vi "_Update Shutting Down.vi"(4 "error in (no error)":errorcluster, 7 "Fault":bool) -> (0 "error Out":errorcluster, 1 "Cancelled":bool, 2 "Error":bool, 3 "InstrState":T1=enum."Fault")   [LabVIEW 2012]
uses:
  Type/_RT Instrument State.ctl
  Type/_LCD Line1 Msg.ctl
  Type/_LCD Line2 Msg.ctl
  Type/_RT LED Num.ctl
  Type/_LED States.ctl
  Type/_Pump Parameter.ctl
  Type/_RW Status.ctl
  _RT Global.vi
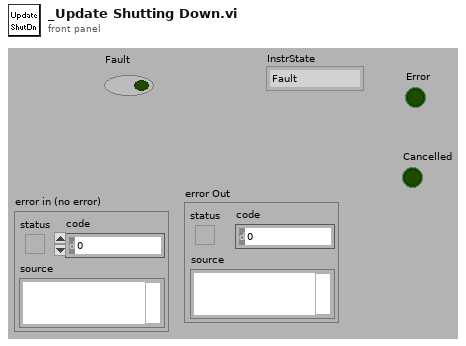
[diagram p1: front panel]
types:
  T1 = typedef "_RT Instrument State.ctl" = enum16{"Initializing", "Mass Spectrometer is Off", "Starting Up", "Turning Power Off", "Going to Standby", "Roughing Pump Ready", "Turning Turbo Off", "Turbo Startup", "Turbopump Ready", "Checking Vacuum", "Going to Ready", "Ready", "Running", "Source Standby", "Lost Communication", "Shutting Down", "Fault", "24V Standby", "Go to 24V Standby", "Turbopump Ready-Waiting"}
  T2 = typedef "_RT LED Num.ctl" = enum8{"ReadKey", "ClearKeyBuffer", "ClearLCD", "BacklightOn"}
  T3 = typedef "_Pump Parameter.ctl" = enum16{"Turn Pump Motor On", "Turn Pump Motor Off", "Read Pump Oil Deficiency", "Read Rotation Switch Point Attained", "Read Ele. Drive Over Temperature", "Read Pump Over Temperature", "Read Set Rotation Speed Attained", "Read Turbopump Accelerates", "Read Actual Rotation Speed in Hz", "Read Motor Current in A", "Read Operating Hours in h", "Read Motor Voltage in V", "Read Motor Power in W", "Set Rotation Speed Switchpoint in %", "Clear Error", "Read Error Code", "Read Bearing Temperature", "Read Hardware Version", "Read Firmware Version", "Read Operating Hours (Drive)", "Read Rotational Speed (rpm)", "Read Power Stage Temperature", "Read Electronics Temperature", "Read Upper Pump Temperature", "Read Motor Temperature", "Read Error Code History, 1", "Read Error Code History, 2", "Read Error Code History, 3", "Read Error Code History, 4", "Read Error Code History, 5", "Read Error Code History, 6", "Read Error Code History, 7", "Read Error Code History, 8", "Read Error Code History, 9", "Read Error Code History, 10"}
  T4 = typedef "_LED States.ctl" = enum8{"Idle", "Solid B", "Solid R", "Solid P", "Off B", "Off R", "Off P", "Off BRP", "Off RP", "Flash R&P", "Flash P"}
  T5 = typedef "_RW Status.ctl" = enum8{"Done", "Do Read", "Do Write", "Set Latch1", "Set Latch2", "Set Latch3", "Set Latch4", "RP ON", "EL ON", "Serial Send", "Set LC Out", "Get LC In", "Read VAC", "Table Test", "Get Interlock", "Do Read2", "Do Write2"}
  T6 = typedef "_LCD Line2 Msg.ctl" = u16
  T7 = typedef "_LCD Line1 Msg.ctl" = u16
  T8 = typedef "_RT Startup Options.ctl" = cluster{"Door":bool, "Curtain":bool, "Pressure":bool, "Turbo":bool, "SysPoll":bool, "GasFlag":bool}
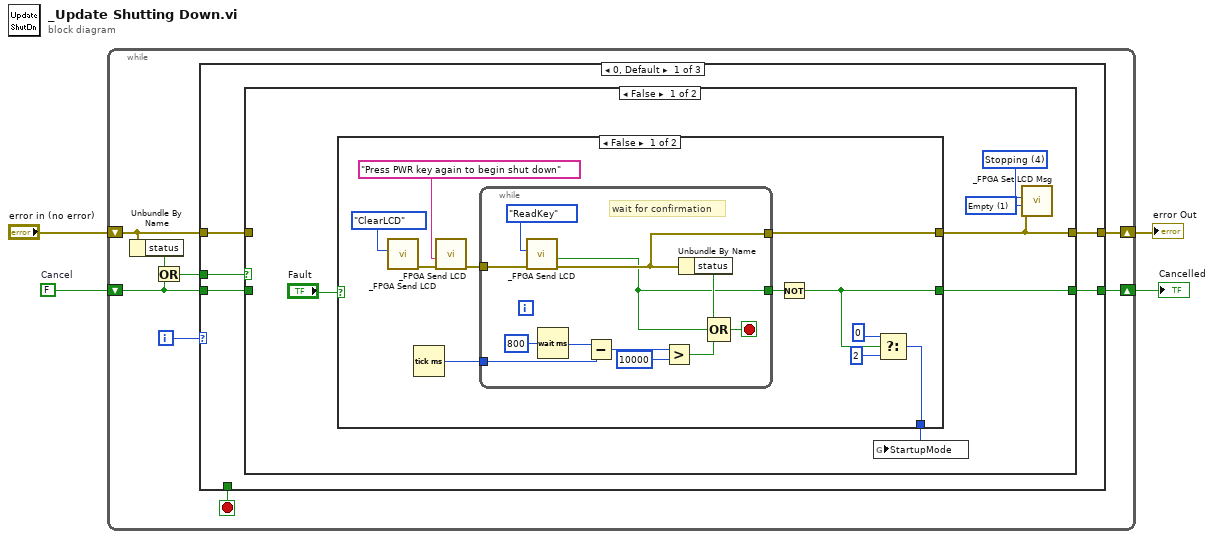
[diagram p0: block diagram]
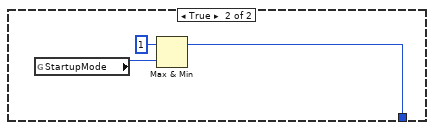
[diagram p2: hidden frame]
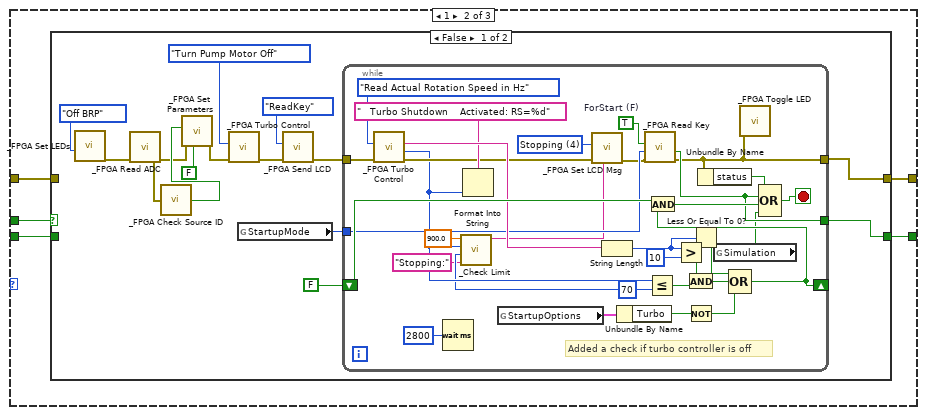
[diagram p4: hidden frame]
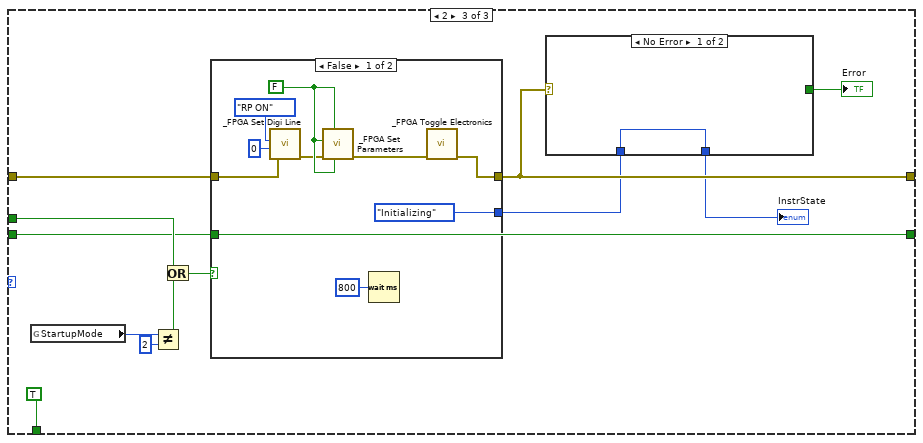
[diagram p6: hidden frame]
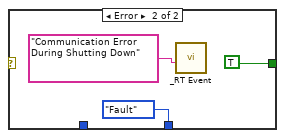
[diagram p7: hidden frame]
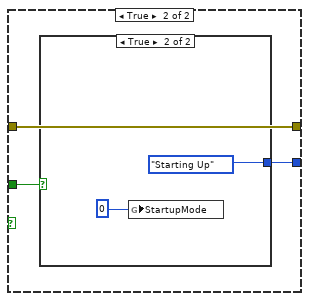
[diagram p8: hidden frame]
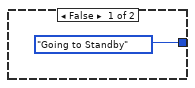
[diagram p9: hidden frame]
diagram:
  w3 = FALSE  # Cancel
  n1 = while {
    shift-right: [w6] -> w2
    shift-left: "error in (no error)" -> [w11]
    shift-right: [w5] -> w1
    shift-left: w3 -> [w10]
    i -> [w8]
    stop <- w7 stop-if-true
    n2 = Unbundle By Name(w11) -> ("status"=w12:bool)
    n3 = Or(x=w12, y=w10) -> (x .or. y?=w9:bool)
    n4 = case shown="0, Default" w8 {
      tunnel: w11 -> [w16 w56 w116]
      tunnel: w10 -> [w14 w54 w105]
      tunnel: w9 -> [w17 w52 w111]
      tunnel: [_ _ TRUE] -> w7
      tunnel: [w15 w55 w114] -> w6
      tunnel: [w13 w53 w105] -> w5
      frame 0, Default {
        n5 = case shown="False" w17 {
          tunnel: w16 -> [_ w51]
          tunnel: [w18 w51] -> w15
          tunnel: w14 -> [_ w50]
          tunnel: [w22 w50] -> w13
          frame False {
            w19 = T6 1 items=["Same", "Empty", "VacFail", "Cancel", "CheckGas", "EleFail", "Probe1Fail", "Probe2Fail", "HeaterFail", "DoorOpen", "CheckComm", "PressStart"] ("Line2Msg (same)")
            w20 = T7 4 items=["Same", "Empty", "Connected", "Starting", "Stopping", "Action", "On", "Service", "Call", "Acquiring", "Source"] ("Line1Msg (same)")
            n6 = case shown="False" "Fault" {
              tunnel: [w33 _] -> w18
              tunnel: [w30 _] -> w22
              tunnel: [w28 w47] -> w21
              frame False {
                n7 = call "_FPGA Send LCD.vi"("Command"=_RT_LED_Num."ClearLCD" ("LED#")) -> ("error out"=w27:errorcluster)  [unwired: 4 in, 3 out]
                n8 = Tick Count (ms)() -> (millisecond timer value=w34:u32)
                n9 = call "_FPGA Send LCD.vi"("error in (no error)"=w27, "Message"="Press PWR key again to begin shut down" ("Command")) -> ("error out"=w25:errorcluster)  [unwired: 3 in, 3 out]
                n10 = while {
                  tunnel: w25 -> [w38]
                  tunnel: [w37] -> w33
                  tunnel: w34 -> [w42]
                  tunnel: [w35] -> w32
                  stop <- w45 stop-if-true
                  # "wait for confirmation"
                  n11 = call "_FPGA Send LCD.vi"("error in (no error)"=w38, "Command"=_RT_LED_Num."ReadKey" ("LED#")) -> ("error out"=w37:errorcluster, "Key Pressed"=w35:bool)  [unwired: 3 in, 2 out]
                  n12 = Wait (ms)(milliseconds to wait=u32 800) -> (millisecond timer value=w43:u32)
                  n13 = Subtract(x=w43, y=w42) -> (x-y=w41:u32)
                  n14 = Greater?(x=w41, y=u32 10000) -> (0:w36:bool)
                  n15 = Unbundle By Name(w37) -> ("status"=w44:bool)
                  n16 = Compound Arithmetic op=OR(w44, w35, w36) -> (w45:bool)
                }
                n17 = Not(x=w32) -> (.not. x?=w30:bool)
                n18 = Select(t=u8 0 ("f"), s=w30, f=u8 2) -> (s? t:f=w28:u8)
              }
              frame True {
                n19 = global read "_RT Global.vi" "StartupMode"() -> (w49:u8)
                n20 = Max & Min(x=u8 1, y=w49) -> (max(x,y)=w47:u8)  [unwired: 1 out]
              }
            }
            n21 = global write "_RT Global.vi" "StartupMode"(w21) -> ()
            n22 = call "_FPGA Set LCD Msg.vi"("error in"=w18, "Line2Msg (same)"=w19, "Line1Msg (same)"=w20) -> ()  [unwired: 4 in, 3 out]
          }
          frame True {
          }
        }
      }
      frame 1 {
        n23 = case shown="False" w52 {
          tunnel: w56 -> [_ w104]
          tunnel: [w67 w104] -> w55
          tunnel: w54 -> [_ w103]
          tunnel: [w66 w103] -> w53
          frame False {
            n24 = call "_FPGA Set LEDs.vi"("LED Command"=_LED_States."Off BRP") -> ("error out"=w61:errorcluster)  [unwired: 3 in, 3 out]
            n25 = call "_FPGA Read ADC.vi"("error in"=w61) -> ("error out"=w62:errorcluster)  [unwired: 1 in, 7 out]
            n26 = call "_FPGA Check Source ID.vi"("error in (no error)"=w62) -> ("Source ID OK"=w63:bool)
            n27 = call "_FPGA Set Parameters.vi"("ExhaustGas (on)"=FALSE, "error in"=w62, "HSID Temp (on)"=w63) -> ("error out"=w57:errorcluster)  [unwired: 6 in, 2 out]
            n28 = call "_FPGA Turbo Control.vi"("error in (no error)"=w57, "Command"=_Pump_Parameter."Turn Pump Motor Off") -> ("error out"=w59:errorcluster)  [unwired: 2 in, 5 out]
            n29 = global read "_RT Global.vi" "StartupMode"() -> (w65:u8)
            n30 = call "_FPGA Send LCD.vi"("error in (no error)"=w59, "Command"=_RT_LED_Num."ReadKey" ("LED#")) -> ("error out"=w58:errorcluster)  [unwired: 3 in, 3 out]
            n31 = while {
              tunnel: [w71] -> w67
              tunnel: w58 -> [w90]
              tunnel: [w89] -> w66
              shift-right: [w84] -> _
              shift-left: FALSE -> [w96]
              tunnel: w65 -> [w88]
              stop <- w98 stop-if-true
              w80 = T7 4 items=["Same", "Empty", "Connected", "Starting", "Stopping", "Action", "On", "Service", "Call", "Acquiring", "Source"] ("Line1Msg (same)")
              w93 = TRUE  # ForStart (F)
              w77 = 70 ("y")
              # "Added a check if turbo controller is off"
              n32 = call "_FPGA Turbo Control.vi"("error in (no error)"=w90, "Command"=_Pump_Parameter."Read Actual Rotation Speed in Hz") -> ("error out"=w86:errorcluster, "Speed"=w78:i32, "Reply"=w91:string)  [unwired: 1 in, 4 out]
              n33 = Wait (ms)(milliseconds to wait=u32 2800) -> ()  [unwired: 1 out]
              n34 = call "_Check Limit.vi"("Header"="Stopping:" ("Header (10Ch)"), "Min (0)"=w77, "Current"=w78, "Max (100)"=900.0) -> ("ProgressBar"=w76:string)  [unwired: 3 out]
              n35 = Format Into String(format string="   Turbo Shutdown    Activated: RS=%d" ("Command"), w78) -> ()  [unwired: 2 in, 2 out]
              n36 = global read "_RT Global.vi" "StartupOptions"() -> (w82:T8)
              n37 = call "_FPGA Set LCD Msg.vi"("Info"=w76, "error in"=w86, "Line1Msg (same)"=w80) -> ("error out"=w85:errorcluster)  [unwired: 4 in, 2 out]
              n38 = String Length(string=w91) -> (length=w73:i32)
              n39 = Unbundle By Name(w82) -> ("Turbo"=w83:bool)
              n40 = call "_FPGA Read Key.vi"("error in (no error)"=w85, "CurStartupMode (0)"=w88, "ForStart (F)"=w93) -> ("error out"=w71:errorcluster, "Key Pressed"=w89:bool)  [unwired: 2 in, 2 out]
              n41 = Less Or Equal?(x=w78, y=w77) -> (x <= y?=w99:bool)
              n42 = Greater?(x=w73, y=10) -> (0:w100:bool)
              n43 = And(x=w100, y=w99) -> (x .and. y?=w97:bool)
              n44 = Not(x=w83) -> (.not. x?=w81:bool)
              n45 = Less Or Equal To 0?(x=w73) -> (x <= 0?=w72:bool)
              n46 = Unbundle By Name(w71) -> ("status"=w94:bool)
              n47 = global read "_RT Global.vi" "Simulation"() -> (w74:bool)
              n48 = Compound Arithmetic op=OR(w72, w97, w81) -> (w84:bool)
              n49 = And(x=w96, y=w84) -> (x .and. y?=w95:bool)
              n50 = call "_FPGA Toggle LED.vi"("error in (no error)"=w71) -> ()  [unwired: 4 in, 4 out]
              n51 = Compound Arithmetic op=OR(w94, w89, w95, w74) -> (w98:bool)
            }
          }
          frame True {
          }
        }
      }
      frame 2 {
        n52 = global read "_RT Global.vi" "StartupMode"() -> (w109:u8)
        n53 = Not Equal?(x=w109, y=u8 2) -> (x != y?=w108:bool)
        n54 = Or(x=w111, y=w108) -> (x .or. y?=w110:bool)
        n55 = case shown="False" w110 {
          tunnel: w116 -> [w127 w132]
          tunnel: [w123 w132] -> w114
          tunnel: [_RT_Instrument_State."Initializing" ("Next InstrState") w131] -> w106
          tunnel: w105 -> [_ w130]
          frame False {
            w124 = FALSE ("CurGas (on)")
            n56 = call "_FPGA Set Digi Line.vi"("error in"=w127, "States"=u16 0, "Line (Set Latch1)"=_RW_Status."RP ON") -> ("error out"=w122:errorcluster)  [unwired: 4 out]
            n57 = call "_FPGA Set Parameters.vi"("ExhaustGas (on)"=w124, "CurGas (on)"=w124, "error in"=w122, "HSID Temp (on)"=w124) -> ("error out"=w121:errorcluster)  [unwired: 5 in, 2 out]
            n58 = Wait (ms)(milliseconds to wait=u32 800) -> ()  [unwired: 1 out]
            n59 = call "_FPGA Toggle Electronics.vi"("error in"=w121) -> ("error out"=w123:errorcluster)  [unwired: 2 in, 5 out]
          }
          frame True {
            n60 = case shown="True" w130 {
              tunnel: [_RT_Instrument_State."Going to Standby" ("Next InstrState") _RT_Instrument_State."Starting Up" ("Next InstrState")] -> w131
              frame False {
              }
              frame True {
                n61 = global write "_RT Global.vi" "StartupMode"(u8 0 ("f")) -> ()
              }
            }
          }
        }
        n62 = case shown="No Error" w114 {
          tunnel: [_ TRUE] -> w113
          tunnel: [w117 _RT_Instrument_State."Fault" ("Next InstrState")] -> w107
          tunnel: w106 -> [w117 _]
          frame No Error {
          }
          frame Error {
            n63 = call "_RT Event.vi"("Event"="Communication Error During Shutting Down") -> ()  [unwired: 2 in, 5 out]
          }
        }
        "Error" <- w113
        "InstrState" <- w107
      }
    }
  }
  "Cancelled" <- w1
  "error Out" <- w2
